vi "Save String Array.vi"(8 "error in (no error)":errorcluster, 9 "Project Folder":path, 10 "Label":string, 11 "Str Array":string[](array[string])) -> (0 "error out":errorcluster)   [LabVIEW 2015]
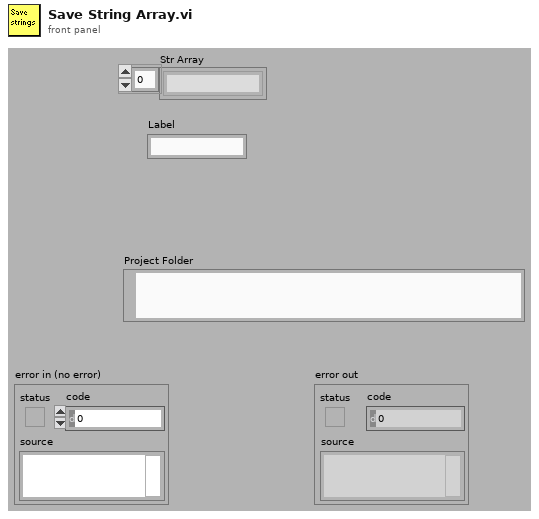
[diagram p1: front panel]
types:
  T1 = enum16{"open", "replace", "create", "open or create", "replace or create", "replace or create with confirmation"}
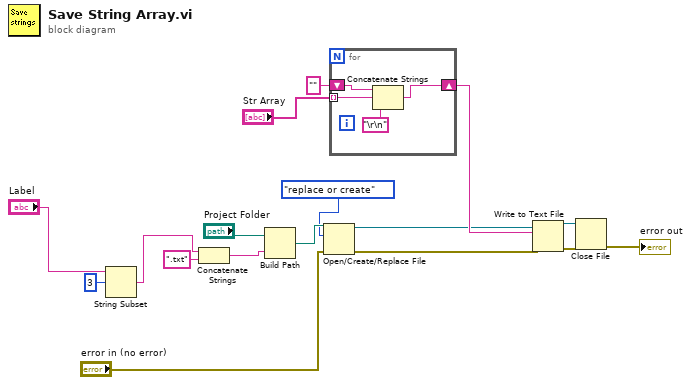
[diagram p0: block diagram]
diagram:
  n1 = String Subset(string="Label", offset (0)=3) -> (substring=w1:string)  [unwired: 1 in]
  n2 = Concatenate Strings(w1, ".txt" ("string")) -> (w11:string)
  n3 = Build Path(base path="Project Folder", name or relative path=w11) -> (appended path=w16:path)
  n4 = Open/Create/Replace File(file path (use dialog)=w16, error in="error in (no error)", operation (0:open)=T1."replace or create") -> (refnum out=w7:refnum<file>, error out=w6:errorcluster)  [unwired: 3 in, 1 out]
  n5 = for {
    shift-right: [w20] -> w8
    shift-left: "" -> [w21]
    tunnel: "Str Array" -> [w19] mode=indexing
    n6 = Concatenate Strings(w21, w19, "\r\n") -> (w20:string)
  }
  n7 = Write to Text File(file (use dialog)=w7, text=w8, error in=w6) -> (refnum out=w13:refnum<file>, error out=w14:errorcluster)  [unwired: 1 in, 1 out]
  n8 = Close File(refnum=w13, error in=w14) -> (error out=→"error out":errorcluster)  [unwired: 1 out]
